vi ";atches_zu_position_und_winkel_mit_text.vi"(11 "Matches (Pattern Matching 1)":T1(array[cluster])) -> (0 "Angle":sgl, 1 "Position":cluster{"x":sgl, "y":sgl}, 2 "x":sgl, 3 "y":sgl, 4 "String":string, 5 "Array":sgl[](array[numeric]), 6 "String 2":string, 7 "String 3":string)   [LabVIEW 2014]
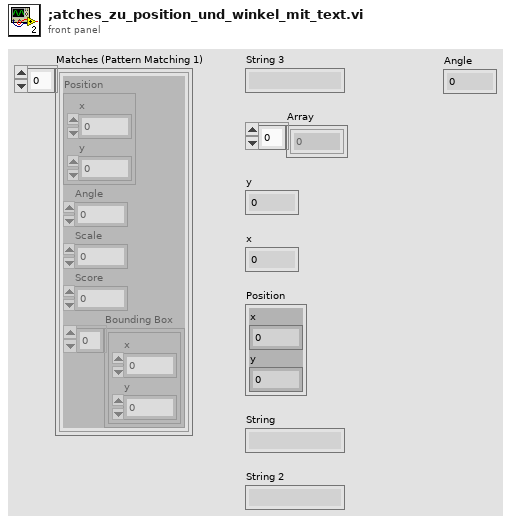
[diagram p1: front panel]
types:
  T1 = cluster{"Position":cluster{"x":sgl, "y":sgl}, "Angle":sgl, "Scale":sgl, "Score":sgl, "Bounding Box":cluster{"x":sgl, "y":sgl}[]}[]
  T2 = cluster{"Matches (Pattern Matching 1)[0]":cluster{"Position":cluster{"x":sgl, "y":sgl}, "Angle":sgl, "Scale":sgl, "Score":sgl, "Bounding Box":cluster{"x":sgl, "y":sgl}[]}, "Matches (Pattern Matching 1)[1]":cluster{"Position":cluster{"x":sgl, "y":sgl}, "Angle":sgl, "Scale":sgl, "Score":sgl, "Bounding Box":cluster{"x":sgl, "y":sgl}[]}, "Matches (Pattern Matching 1)[2]":cluster{"Position":cluster{"x":sgl, "y":sgl}, "Angle":sgl, "Scale":sgl, "Score":sgl, "Bounding Box":cluster{"x":sgl, "y":sgl}[]}, "Matches (Pattern Matching 1)[3]":cluster{"Position":cluster{"x":sgl, "y":sgl}, "Angle":sgl, "Scale":sgl, "Score":sgl, "Bounding Box":cluster{"x":sgl, "y":sgl}[]}, "Matches (Pattern Matching 1)[4]":cluster{"Position":cluster{"x":sgl, "y":sgl}, "Angle":sgl, "Scale":sgl, "Score":sgl, "Bounding Box":cluster{"x":sgl, "y":sgl}[]}, "Matches (Pattern Matching 1)[5]":cluster{"Position":cluster{"x":sgl, "y":sgl}, "Angle":sgl, "Scale":sgl, "Score":sgl, "Bounding Box":cluster{"x":sgl, "y":sgl}[]}, "Matches (Pattern Matching 1)[6]":cluster{"Position":cluster{"x":sgl, "y":sgl}, "Angle":sgl, "Scale":sgl, "Score":sgl, "Bounding Box":cluster{"x":sgl, "y":sgl}[]}, "Matches (Pattern Matching 1)[7]":cluster{"Position":cluster{"x":sgl, "y":sgl}, "Angle":sgl, "Scale":sgl, "Score":sgl, "Bounding Box":cluster{"x":sgl, "y":sgl}[]}, "Matches (Pattern Matching 1)[8]":cluster{"Position":cluster{"x":sgl, "y":sgl}, "Angle":sgl, "Scale":sgl, "Score":sgl, "Bounding Box":cluster{"x":sgl, "y":sgl}[]}}
  T3 = cluster{"Position":cluster{"x":sgl, "y":sgl}, "Angle":sgl, "Scale":sgl, "Score":sgl, "Bounding Box":cluster{"x":sgl, "y":sgl}[]}
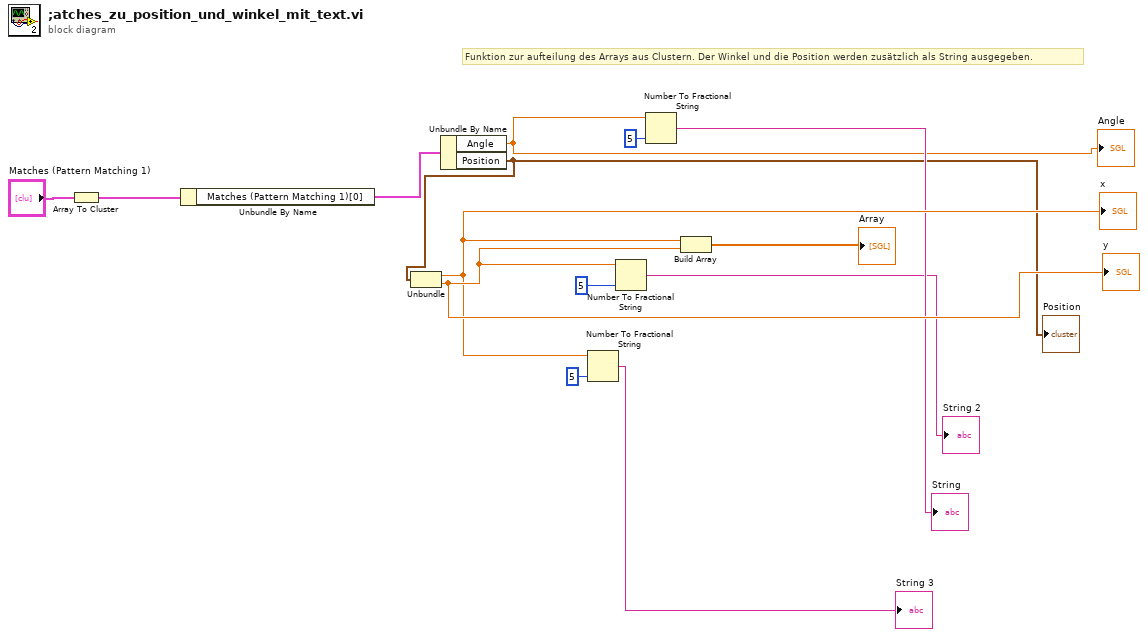
[diagram p0: block diagram]
diagram:
  # "Funktion zur aufteilung des Arrays aus Clustern. Der Winkel und die Position werden zusätzlich als String ausgegeben."
  n1 = Array To Cluster(array="Matches (Pattern Matching 1)") -> (cluster=w7:T2)
  n2 = Unbundle By Name(w7) -> ("Matches (Pattern Matching 1)[0]"=w6:T3)
  n3 = Unbundle By Name(w6) -> ("Angle"=w4:sgl, "Position"=w8:cluster{"x":sgl, "y":sgl})
  "Position" <- w8
  "Angle" <- w4
  n4 = Unbundle(w8) -> ("x"=w13:sgl, "y"=w14:sgl)
  "y" <- w14
  "x" <- w13
  n5 = Number To Fractional String(number=w13, precision (6)=i16 5) -> (F-format string=→"String 3":string)  [unwired: 2 in]
  n6 = Number To Fractional String(number=w14, precision (6)=i16 5) -> (F-format string=→"String 2":string)  [unwired: 2 in]
  n7 = Number To Fractional String(number=w4, precision (6)=i16 5) -> (F-format string=→"String":string)  [unwired: 2 in]
  n8 = Build Array(w13, w14) -> (→"Array":sgl[])
